vi "CALC_MARK_REF_X.vi"(0 "VISA IN":refnum<visa-resource-name>, 1 "X-axis Value":i32, 5 "error in":errorcluster, 7 "Channel":i32) -> (14 "VISA Out":refnum<visa-resource-name>, 19 "error out":errorcluster)   [LabVIEW 2018, in "PNA-X.lvlib"]
doc: "CALCulate<cnum>:MARKer:REFerence:X <num> \n(Read-Write) Sets and returns the absolute x-axis value of the reference marker (marker 10). \nSee Critical Note \n<cnum> Channel number of the measurement. There must be a selected measurement \non that channel. If unspecified, <cnum> is set to 1. \n<num> X-axis value. Choose any number within the operating domain of the reference \nmarker. \nExamples CALC:MARK:REF:X 1e9 \ncalculate2:marker:reference:x 1e6 \nQuery Syntax CALCulate<cnum>:MARKer:REFerence:X? \nReturn Type Numeric \n1539\n\nDefault If the first Marker, turns ON in the middle of the X-axis span. If not, turns ON \nat the position of the active marker."
uses:
  PNA-X.lvlib
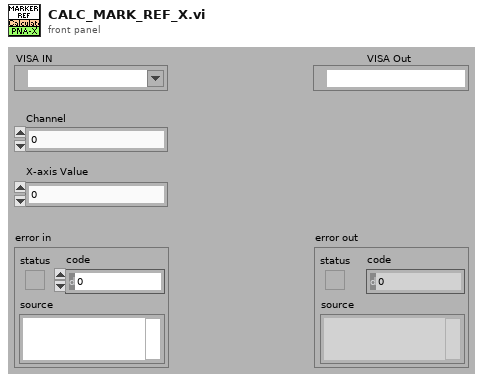
[diagram p1: front panel]
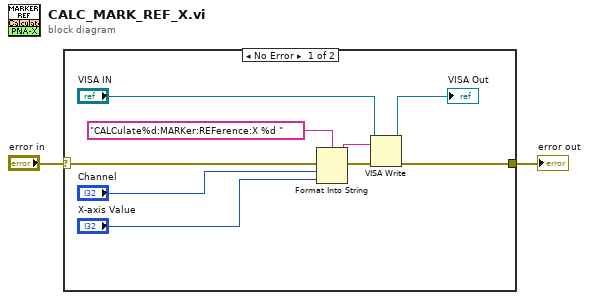
[diagram p0: block diagram]
diagram:
  n1 = case shown="No Error" "error in" {
    selector: "error in" -> [w11 w12]
    tunnel: [w6 w12] -> w1
    frame No Error {
      n2 = Format Into String(format string="CALCulate%d:MARKer:REFerence:X %d " ("Cmdline"), error in=w11, "Channel", "X-axis Value") -> (resulting string=w9:string, error out=w10:errorcluster)  [unwired: 1 in]
      n3 = VISA Write(VISA resource name="VISA IN", write buffer=w9, error in (no error)=w10) -> (VISA resource name out=→"VISA Out":refnum<visa-resource-name>, error out=w6:errorcluster)  [unwired: 1 out]
    }
    frame Error {
    }
  }
  "error out" <- w1
